vi "QueryInProgress.vi"(8 "error in (no error)":errorcluster, 11 "Action":enum16{"Get", "Set False", "Set True"}(ring)) -> (0 "error out":errorcluster, 3 "Value":bool)   [LabVIEW 2020, in "plugin_flodx_pressure.lvlib" / "plugin.lvlib" / "Instrument Manager.lvlib"]
doc: "FGV (Function Global Variable) to keep track of the Query state, used\nin the Instrument Manager Loop to control race conditions."
uses:
  Instrument Manager.lvlib
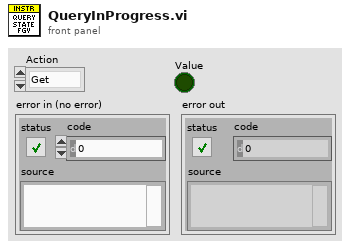
[diagram p1: front panel]
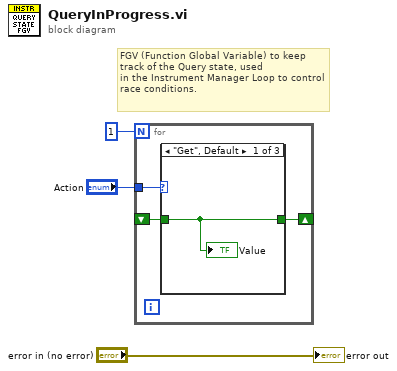
[diagram p0: block diagram]
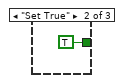
[diagram p2: hidden frame]
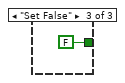
[diagram p3: hidden frame]
diagram:
  # "FGV (Function Global Variable) to keep track of the Query state, used\nin the Instrument Manager Loop to control race conditions."
  n1 = for {
    N: 1 -> [_]
    tunnel: "Action" -> [w6]
    shift-right: [w4] -> _
    shift-left: _ -> [w5]
    n2 = case shown="\"Get\", Default" w6 {
      tunnel: w5 -> [w7 _ _]
      tunnel: [w7 TRUE FALSE] -> w4
      frame "Get", Default {
        "Value" <- w7
      }
      frame "Set True" {
      }
      frame "Set False" {
      }
    }
  }
  "error out" <- "error in (no error)"
